vi "Wrap Position.vi"(11 "Movable in":refnum<class "Element.lvclass">) -> (3 "Movable out":refnum<class "Element.lvclass">)   [LabVIEW 2021, in "Element.lvclass"]
uses:
  Element.lvclass
  Element.lvclass/Element.ctl
  Motion/Motion.lvclass
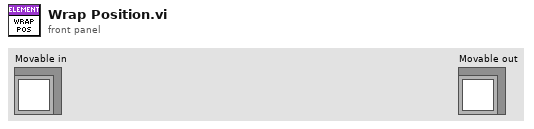
[diagram p1: front panel]
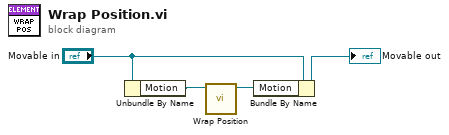
[diagram p0: block diagram]
diagram:
  n1 = Unbundle By Name("Movable in") -> ("Motion"=w4:refnum<class "Motion.lvclass">)
  n2 = call "Wrap Position.vi"("Motion in"=w4) -> ("Motion out"=w2:refnum<class "Motion.lvclass">)  [unwired: 10 in]
  n3 = Bundle By Name(cluster="Movable in", "Motion"=w2) -> (→"Movable out":refnum<class "Element.lvclass">)
